vi "SQL_Find Item.vi"(6 "index":i32, 7 "Column to Sort":i32, 8 "error in (no error)":errorcluster, 9 "Element":string, 10 "Table":string, 11 "SQL in":refnum<class "SQL.lvclass">) -> (0 "error out":errorcluster, 1 "Element":string, 2 "RowData":string[](array[string]), 3 "SQL out":refnum<class "SQL.lvclass">)   [LabVIEW 2012, in "SQL.lvclass"]
uses:
  SQL.lvclass
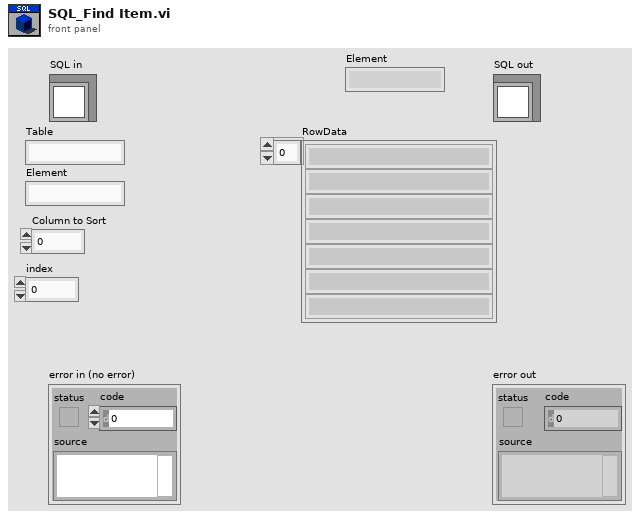
[diagram p1: front panel]
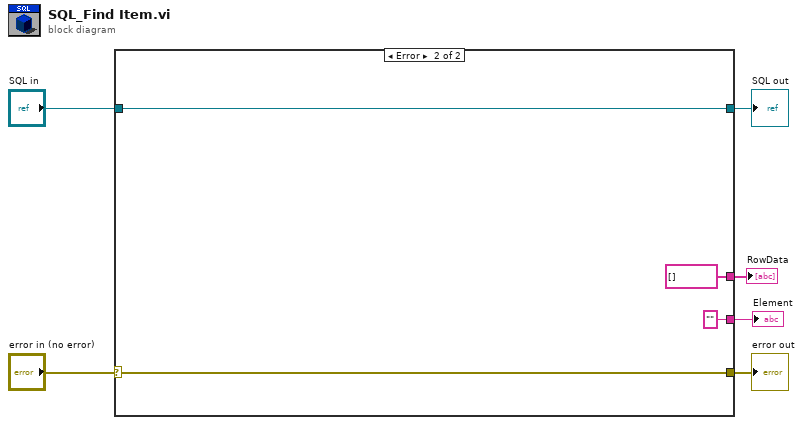
[diagram p0: block diagram]
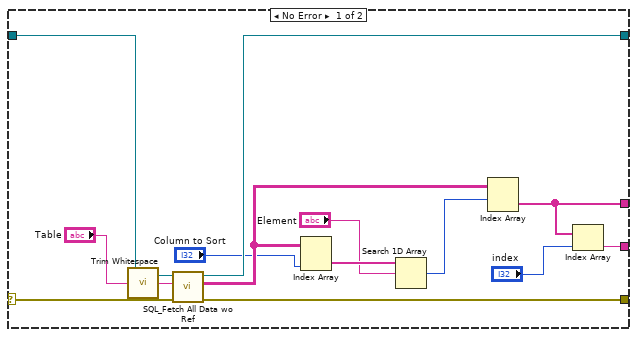
[diagram p2: hidden frame]
diagram:
  n1 = case shown="Error" "error in (no error)" {
    selector: "error in (no error)" -> [w20 w24]
    tunnel: [w19 w24] -> w5
    tunnel: [w16 w23] -> w3
    tunnel: "SQL in" -> [w17 w23]
    tunnel: [w9 string[] [] ("InitialData")] -> w2
    tunnel: [w7 "" ("data")] -> w1
    frame No Error {
      n2 = call <vilib>:"Trim Whitespace.vi"("string"="Table") -> ("trimmed string"=w11:string)  [unwired: 1 in]
      n3 = call-dynamic "SQL_Fetch All Data wo Ref.vi"("error in (no error)"=w20, "Table"=w11, "SQL in"=w17) -> ("error out"=w19:errorcluster, "InitialData"=w14:string[][], "SQL out"=w16:refnum<class "SQL.lvclass">)  [unwired: 5 in, 1 out]
      n4 = Index Array(array=w14, index (col)="Column to Sort") -> (element=w15:string[])  [unwired: 1 in]
      n5 = Search 1D Array(1D array=w15, element="Element") -> (index of element=w13:i32)  [unwired: 1 in]
      n6 = Index Array(array=w14, index (row)=w13) -> (element=w9:string[])  [unwired: 1 in]
      n7 = Index Array(array=w9, index="index") -> (element=w7:string)
    }
    frame Error {
    }
  }
  "error out" <- w5
  "SQL out" <- w3
  "RowData" <- w2
  "Element" <- w1
